vi "Calculate Hysteresis.vi"(0 "trigger source":u8, 1 "actual channel configuration":T1[](array[typedef]) {"vertical offset" format="%_3p"; "vertical range" format="%_3p"}, 5 "trigger slope":T5, 7 "level (V)":dbl, 9 "hysteresis (V)":dbl, 11 "error in":errorcluster) -> (4 "high level (V)":dbl, 6 "low level (V)":dbl, 15 "error out":errorcluster)   [LabVIEW 2015, in "Device Session.lvclass"]
doc: "Computes the hysteresis for the edge trigger. This VI will return an error if <B>hysteresis (V)</B> is a negative value.\n\n<B>Input Parameters</B>\n\n<B>actual channel configuration</B> is an array of configurations for all channels, including the channel selected to compute hysteresis for.\n\n<B>actual channel configuration.channel</B> is the channel that was configured.\n\n<B>actual channel configuration.coupling</B> is the coupling configuration applied to the channel.\n\n'DC': Direct Current coupling.\n'AC': Alternating Current coupling.\n\n<B>actual channel configuration.impedance</B> is the impedance configuration applied to the channel.\n\n'1 mega ohm': The channel was configured with 1 MOhm of impedance.\n'50 ohm': The channel was configured with 50 Ohms of impedance.\n\n<B>actual channel configuration.bandwidth</B> is the coerced bandwidth configuration applied to the channel.\n\n'Full Bandwidth': No attenuation of the signal.\n'Anti-alias Filter': Attenuates unwanted high-frequency signals of an analog signal prior to its conversion into a digital value. These signals would otherwise appear as undesired, aliased frequency components.\n\n<B>actual channel configuration.vertical range</B> is the coerced input range applied to the channel.\n\n<B>actual channel configuration.vertical offset</B> is the coerced vertical offset configuration applied to the channel.\n\n<B>trigger source</B> is the channel to be used as the trigger source.\n\n<B>trigger slope</B> specifies whether the device should trigger on a rising edge or a falling edge.\n\n<B>level (V)</B> specifies the voltage threshold for the trigger.\n\n<B>hysteresis (V)</B> specifies the size of the hysteresis window above or below the specified 'level'. The device triggers when the 'trigger source' signal passes through the 'hysteresis level' you specify with this parameter, has the specified 'trigger slope', and passes through the specified 'level'.\n\n<B>Output Parameters</B>\n\n<B>high level (V)</B> returns the trigger high level calculated using the level, hysteresis level and the trigger slope.\n\n<B>low level (V)</B> returns the trigger low level calculated using the level, hysteresis level and the trigger slope.\n\n<B>error out</B> contains error information. This output provides standard 'error out' functionality."
uses:
  Device Session.lvclass
  <instrlib>/_niInstr/Data Trigger/v1/Shared/Public/Edge Configuration Trigger Slope.ctl
  <instrlib>/HSAI-RIO/Types/v1/Host/Typedefs/Channel Configuration.ctl
  <instrlib>/HSAI-RIO/Types/v1/Host/Typedefs/Coupling.ctl
  <instrlib>/HSAI-RIO/Types/v1/Host/Typedefs/Impedance.ctl
  <instrlib>/HSAI-RIO/Types/v1/Host/Typedefs/Bandwidth.ctl
  <vilib>/Utility/error.llb/Error Cluster From Error Code.vi
  <vilib>/ErrorRing/Error Ring.xnode
  <instrlib>/_niInstr/Data Trigger/v1/Shared/niInstr Data Trigger v1 Shared.lvlib
  <instrlib>/HSAI-RIO/Types/v1/Host/niHSAI Types v1 Host.lvlib
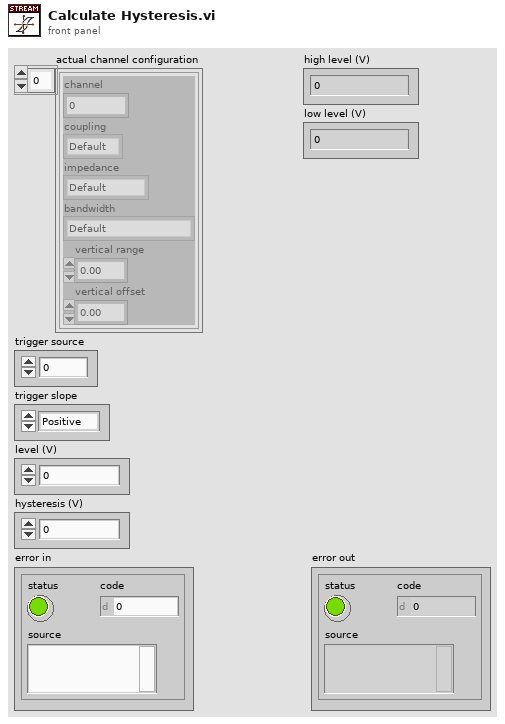
[diagram p1: front panel]
types:
  T1 = typedef "niHSAI Types v1 Host.lvlib/Channel Configuration.ctl" = cluster{"channel":u32, "coupling":T2, "impedance":T3, "bandwidth":T4, "vertical range":dbl, "vertical offset":dbl}
  T2 = typedef "niHSAI Types v1 Host.lvlib/Coupling.ctl" = enum8{"Default", "DC", "AC"}
  T3 = typedef "niHSAI Types v1 Host.lvlib/Impedance.ctl" = enum8{"Default", "1 mega ohm", "50 ohm"}
  T4 = typedef "niHSAI Types v1 Host.lvlib/Bandwidth.ctl" = enum8{"Default", "Full Bandwidth", "Anti-alias Filter"}
  T5 = typedef "niInstr Data Trigger v1 Shared.lvlib/Edge Configuration Trigger Slope.ctl" = enum8{"Positive", "Negative"}
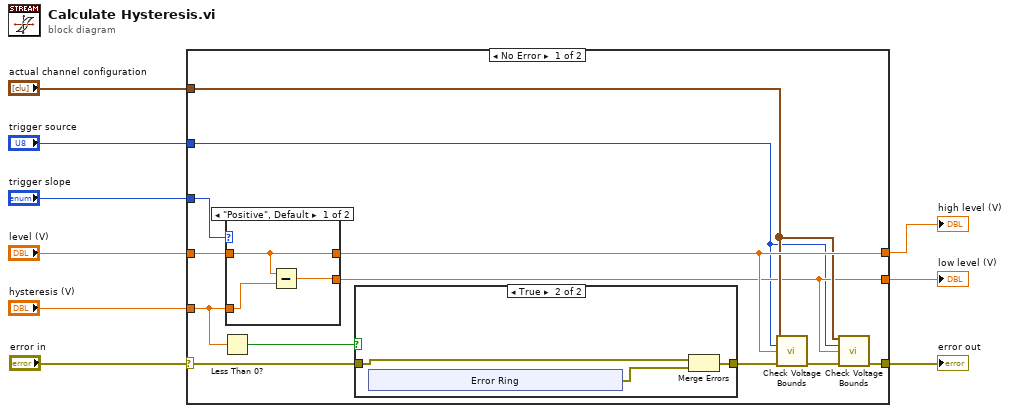
[diagram p0: block diagram]
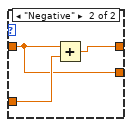
[diagram p3: hidden frame]
diagram:
  n1 = case shown="No Error" "error in" {
    selector: "error in" -> [w15 w36]
    tunnel: "actual channel configuration" -> [w12 _]
    tunnel: "trigger source" -> [w10 _]
    tunnel: "trigger slope" -> [w21 _]
    tunnel: "level (V)" -> [w20 _]
    tunnel: "hysteresis (V)" -> [w19 _]
    tunnel: [w13 w36] -> w3
    tunnel: [w16 _] -> w2
    tunnel: [w11 _] -> w1
    frame No Error {
      n2 = Less Than 0?(x=w19) -> (x < 0?=w18:bool)
      n3 = case shown="\"Positive\", Default" w21 {
        tunnel: w19 -> [w32 w35]
        tunnel: w20 -> [w31 w33]
        tunnel: [w31 w34] -> w16
        tunnel: [w30 w33] -> w11
        frame "Positive", Default {
          n4 = Subtract(x=w31, y=w32) -> (x-y=w30:dbl)
        }
        frame "Negative" {
          n5 = Add(x=w33, y=w35) -> (x+y=w34:dbl)
        }
      }
      n6 = case shown="True" w18 {
        tunnel: [w22 w25] -> w17
        tunnel: w15 -> [w22 w24]
        frame False {
        }
        frame True {
          n7 = xnode "Error Ring"() -> ("error out"=w23:errorcluster)
          n8 = Merge Errors(w24, w23) -> (w25:errorcluster)
        }
      }
      n9 = call "Check Voltage Bounds.vi"("channel configuration"=w12, "trigger source"=w10, "level (V)"=w16, "error in"=w17) -> ("error out"=w14:errorcluster)  [unwired: 11 in]
      n10 = call "Check Voltage Bounds.vi"("channel configuration"=w12, "trigger source"=w10, "level (V)"=w11, "error in"=w14) -> ("error out"=w13:errorcluster)  [unwired: 11 in]
    }
    frame Error {
    }
  }
  "error out" <- w3
  "high level (V)" <- w2
  "low level (V)" <- w1
